vi "UdsRead.vi"(5 "LogSuspend":bool, 7 "TimeoutMs":u32, 8 "error in":errorcluster {"code" format="%.0x"}, 11 "UdsHandleIn":T1) -> (0 "error out":errorcluster {"code" format="%.0x"}, 1 "Data":u8[](array[numeric]) format="%02x", 3 "UdsHandleOut":T1)   [LabVIEW 2011, in "Konvolucio MUDS150628.lvlib"]
uses:
  <instrlib>/Konvolucio MUDS150628/Konvolucio MUDS150628.lvlib
  <instrlib>/Konvolucio MUDS150628/Types/UdsHandleType.ctl
  <instrlib>/Konvolucio MCAN120803/Types/MCanHandleType.ctl
  C:/Program Files/National Instruments/LabVIEW 2011/instr.lib/Konvolucio MCAN120803/Private/Konvolucio.MCAN120803.dll
  Konvolucio MCAN120803/Private/Konvolucio.MCAN120803.dll
  <instrlib>/Konvolucio MUDS150628/Private/UdsLogErrorCheckPoint.vi
  <instrlib>/Konvolucio MCAN120803/Public/Attributes/AttrGetRxPendingMsg.vi
  <instrlib>/Konvolucio MUDS150628/Private/UdsLogCanRxMessage.vi
  <instrlib>/Konvolucio MCAN120803/Konvolucio MCAN120803.lvlib
panel:
  out "LoopCnt":i32
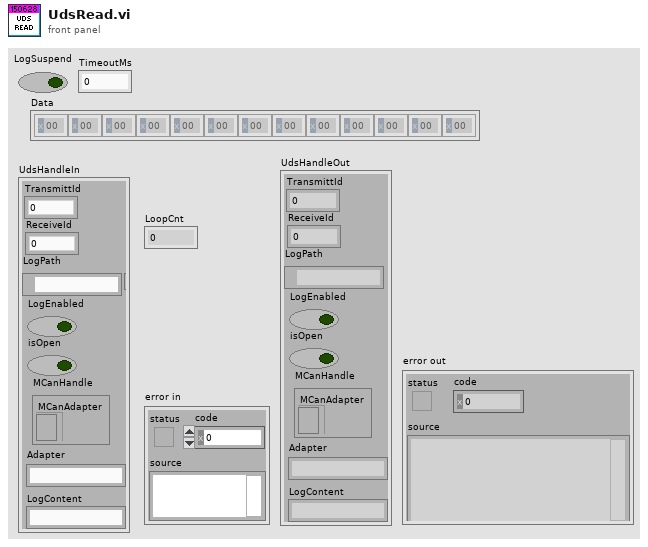
[diagram p1: front panel]
types:
  T1 = typedef "Konvolucio MUDS150628.lvlib/UdsHandleType.ctl" = cluster{"LogPath":path, "LogEnabled":bool, "isOpen":bool, "LogContent":string, "Adapter":string, "MCanHandle":T2, "TransmittId":u32, "ReceiveId":u32}
  T2 = typedef "Konvolucio MCAN120803.lvlib/MCanHandleType.ctl" = cluster{"MCanAdapter":refnum<k24>}
  T3 = typedef "Konvolucio MCAN120803.lvlib/MessageType.ctl" = cluster{"TimeStamp":timestamp, "ArbitrationId":u32, "IsRemote":u8, "DataLength":u8, "Data":u8[]}
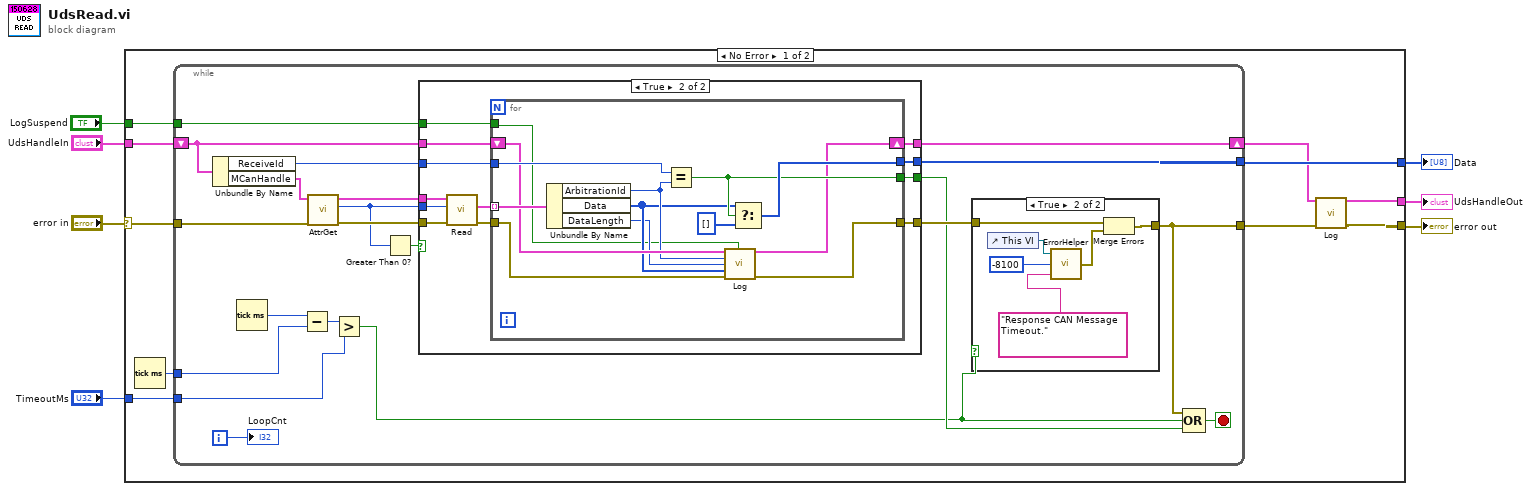
[diagram p0: block diagram]
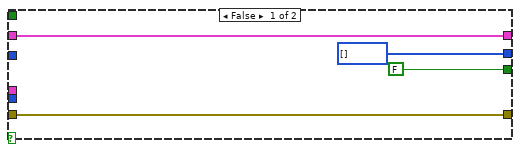
[diagram p3: hidden frame]
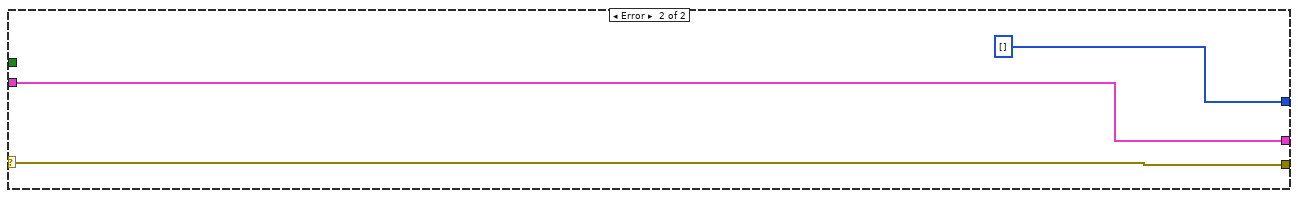
[diagram p4: hidden frame]
diagram:
  n1 = case shown="No Error" "error in" {
    selector: "error in" -> [w16 w75]
    tunnel: "TimeoutMs" -> [w17 _]
    tunnel: [w14 u8[] [] ("Data")] -> w6
    tunnel: [w11 w75] -> w7
    tunnel: "UdsHandleIn" -> [w8 w76]
    tunnel: [w9 w76] -> w3
    tunnel: "LogSuspend" -> [w13 _]
    frame No Error {
      n2 = Tick Count (ms)() -> (millisecond timer value=w15:u32)
      n3 = while {
        tunnel: w17 -> [w21]
        tunnel: w16 -> [w35]
        tunnel: [w28] -> w12
        tunnel: [w30] -> w14
        tunnel: w15 -> [w23]
        tunnel: w13 -> [w19]
        shift-right: [w18] -> w10
        shift-left: w8 -> [w20]
        i -> [w24]
        stop <- w36 stop-if-true
        n4 = Unbundle By Name(w20) -> ("ReceiveId"=w31:u32, "MCanHandle"=w29:T2)
        n5 = Tick Count (ms)() -> (millisecond timer value=w26:u32)
        n6 = Subtract(x=w26, y=w23) -> (x-y=w25:u32)
        n7 = call-poly <instrlib>:"AttrGet.vi"("error in"=w35, "MCanHandleIn"=w29) -> ("error out"=w34:errorcluster, "Value"=w33:i32, "MCanHandleOut"=w32:T2)  [unwired: 7 in]
        n8 = Greater?(x=w25, y=w21) -> (0:w22:bool)
        n9 = Greater Than 0?(x=w33) -> (x > 0?=w37:bool)
        n10 = case shown="True" w37 {
          tunnel: [w49 w57] -> w38
          tunnel: w33 -> [_ w60]
          tunnel: w34 -> [w49 w61]
          tunnel: w32 -> [_ w59]
          tunnel: w31 -> [_ w55]
          tunnel: [u8[] [] ("f") w54] -> w30
          tunnel: [FALSE w53] -> w27
          tunnel: w20 -> [w46 w52]
          tunnel: w19 -> [_ w51]
          tunnel: [w46 w50] -> w18
          frame False {
          }
          frame True {
            n11 = call <instrlib>:"Read.vi"("error in"=w61, "Request Number of Message"=w60, "MCanHandleIn"=w59) -> ("error out"=w58:errorcluster, "Messages"=w56:T3[])  [unwired: 6 in, 1 out]
            n12 = for {
              tunnel: w58 -> [w69]
              tunnel: [w62] -> w57
              tunnel: w56 -> [w74] mode=indexing
              tunnel: w55 -> [w73]
              tunnel: [w72] -> w54
              tunnel: [w70] -> w53
              shift-right: [w64] -> w50
              shift-left: w52 -> [w68]
              tunnel: w51 -> [w63]
              n13 = Unbundle By Name(w74) -> ("ArbitrationId"=w67:u32, "Data"=w66:u8[], "DataLength"=w65:u8)
              n14 = Equal?(x=w73, y=w67) -> (x = y?=w70:bool)
              n15 = call-poly <instrlib>:"Log.vi"("UdsHandleIn"=w68, "LogSuspend"=w63, "Id"=w67, "DataLength"=w65, "Data"=w66, "error in"=w69) -> ("UdsHandleOut"=w64:T1, "error out"=w62:errorcluster)  [unwired: 8 in]
              n16 = Select(t=w66, s=w70, f=u8[] []) -> (s? t:f=w72:u8[])
            }
          }
        }
        n17 = case shown="True" w22 {
          tunnel: w38 -> [w39 w45]
          tunnel: [w39 w44] -> w28
          frame False {
          }
          frame True {
            n18 = control-ref of="This VI"() -> (w43:refnum<vi>)
            n19 = call <instrlib>:"ErrorHelper.vi"("Message"="Response CAN Message Timeout.", "Code"=-8100 ("code"), "This VI"=w43) -> ("error out"=w42:errorcluster)
            n20 = Merge Errors(w45, w42) -> (w44:errorcluster)
          }
        }
        n21 = Compound Arithmetic op=OR(w28, w22, w27) -> (w36:bool)
        "LoopCnt" <- w24
      }
      n22 = call-poly <instrlib>:"Log.vi"("UdsHandleIn"=w10, "error in"=w12) -> ("UdsHandleOut"=w9:T1, "error out"=w11:errorcluster)  [unwired: 12 in]
    }
    frame Error {
    }
  }
  "Data" <- w6
  "error out" <- w7
  "UdsHandleOut" <- w3
